vi "solar_read ThisLogIgnore.vi"(8 "error in (no error)":errorcluster, 11 "solar in":refnum<class "solar.lvclass">) -> (0 "error out":errorcluster, 2 "LogIgnore":string[](array[string]), 3 "solar out":refnum<class "solar.lvclass">)   [LabVIEW 2018, in "solar.lvclass"]
doc: "This returns the messages to ignore while logging. This is useful to avoid uneccessary entries in the SOLAR logs. Use wildcards as astricks ('*'). Messages are case insensitive.\n - 'MyCMD*' - ignores all messages that start with 'MyCMD'\n - '*' - ignores all commands"
uses:
  solar.lvclass
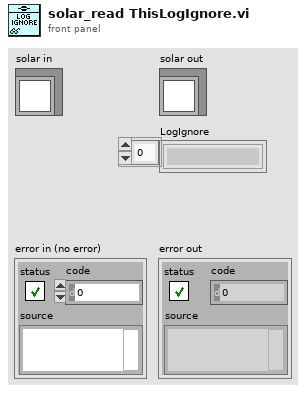
[diagram p1: front panel]
types:
  T1 = typedef "solar_ctl SOLAR Refnum.ctl" = refnum<k1>
  T2 = typedef "solar_ctl SOLAR Global.ctl" = cluster{"Targets":T3[], "AppDir":path, "solar.ini":path, "ConfigsDir":path, "CosmosDir":path, "LogsDir":path, "ExePath":path, "ExeVersion":string, "PartNum":string, "AppSetup":string, "Title":string, "Main.ini":path, "Temp.ini":path, "vSOLAR":string, "Splash.png":string, "SplashWait":i32, "SOLARUE":refnum<user-event>, "VoyagerRefnum":T4, "QTimerRefnum":T5}
  T3 = typedef "solar_ctl Target Global.ctl" = cluster{"Target":string, "Q":refnum<queue>, "UE":refnum<user-event>, "VI":refnum<vi>, "Menu":refnum<k9>, "Data":refnum<data-value>, "Attributes":variant}
  T4 = typedef "solar_voy_ctl Voyager Refnum.ctl" = refnum<k1>
  T5 = typedef "solar_qtimer_ctl Refnum.ctl" = refnum<k1>
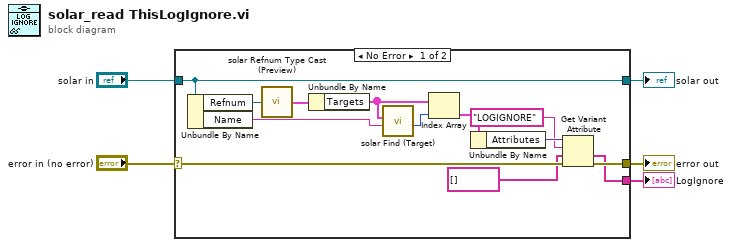
[diagram p0: block diagram]
diagram:
  n1 = case shown="No Error" "error in (no error)" {
    selector: "error in (no error)" -> [w17 w20]
    tunnel: "solar in" -> [w18 w19]
    tunnel: [w9 w20] -> w2
    tunnel: [w18 w19] -> w3
    tunnel: [w8 _] -> w1
    frame No Error {
      n2 = Unbundle By Name(w18) -> ("Refnum"=w13:T1, "Name"=w16:string)
      n3 = call "solar Refnum Type Cast (Preview).vi"("Refnum"=w13) -> ("SOLAR"=w12:T2)  [unwired: 8 in]
      n4 = Unbundle By Name(w12) -> ("Targets"=w14:T3[])
      n5 = call "solar Find (Target).vi"("Target"=w16, "Targets"=w14) -> ("Target Index"=w15:i32)  [unwired: 8 in, 1 out]
      n6 = Index Array(array=w14, index=w15) -> (element=w11:T3)
      n7 = Unbundle By Name(w11) -> ("Attributes"=w10:variant)
      n8 = Get Variant Attribute(Variant=w10, name="LOGIGNORE", default value (empty Variant)=string[] [] ("Ctrls"), error in=w17) -> (value=w8:string[], error out=w9:errorcluster)  [unwired: 2 out]
    }
    frame Error {
    }
  }
  "error out" <- w2
  "solar out" <- w3
  "LogIgnore" <- w1
